vi "SubVI_SaveWaveform.vi"(8 "frequency":i32, 9 "Path":string, 11 "VISA resource name":refnum<visa-resource-name>) -> (3 "VISA resource name out":refnum<visa-resource-name>)   [LabVIEW 2021]
uses:
  <vilib>/Waveform/WDTFileIO.llb/Export Waveform To Spreadsheet File.vi
panel:
  out "Waveform Graph":waveform(dbl)(graph)
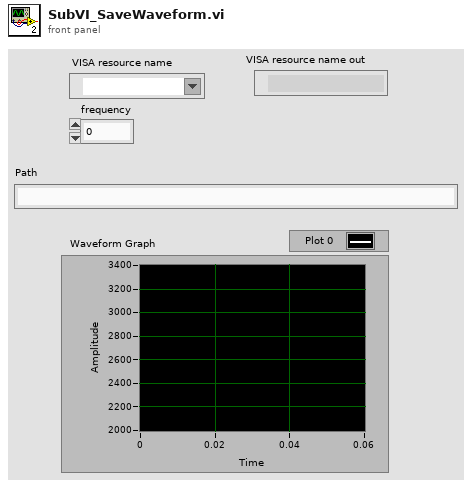
[diagram p1: front panel]
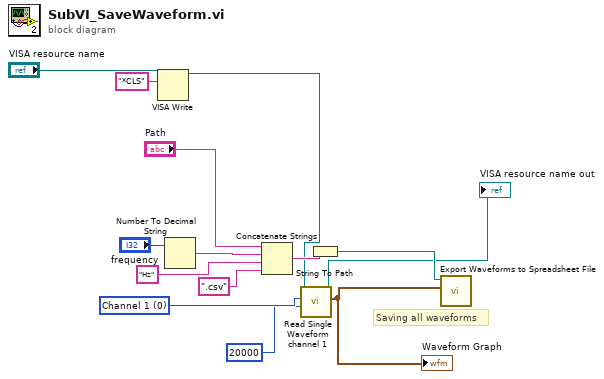
[diagram p0: block diagram]
diagram:
  w8 = u16 0 items=["Channel 1", "Channel 2", "Channel 3", "Channel 4", "Math"] ("Source (0: Channel 1)")
  # "Saving all waveforms"
  n1 = VISA Write(VISA resource name="VISA resource name", write buffer="*CLS") -> (VISA resource name out=w2:refnum<visa-resource-name>)  [unwired: 1 in, 2 out]
  n2 = Number To Decimal String(number="frequency") -> (decimal integer string=w13:string)  [unwired: 1 in]
  n3 = Concatenate Strings("Path", w13, "Hz" ("string"), ".csv" ("string")) -> (w12:string)
  n4 = call "Read Single Waveform channel 1.vi"("Timeout (10000 ms)"=u32 20000, "Source (0: Channel 1)"=w8, "VISA resource name"=w2) -> ("Waveform Data"=w6:waveform(dbl), "VISA resource name out"=→"VISA resource name out":refnum<visa-resource-name>)  [unwired: 6 in, 1 out]
  "Waveform Graph" <- w6
  n5 = String To Path(string=w12) -> (path=w14:path)
  n6 = call-poly <vilib>:"Export Waveforms to Spreadsheet File.vi"("waveform"=w6, "file path (dialog if empty)"=w14) -> ()  [unwired: 8 in, 2 out]
